vi "Dialog_Confirm Tling Parameters.vi"(0 "x FOV":dbl format="%#_3p", 5 "y FOV":dbl format="%#_3p", 9 "actual \noverlap\npercentage":dbl format="%#_3g", 11 "Error In":errorcluster, 12 "Tiling Rows":dbl, 13 "Tiling Columns":dbl) -> (6 "Cancelled?":bool, 15 "Error Out":errorcluster)   [LabVIEW 2012]
doc: "SciScan 1.2 160622\nThis VI has no controls.\nThis is a dummy whihc runs when user selects a macro command which does not require any arguments"
panel:
  in  "Cancel Button":bool
  in  "OK Button":bool
  # "Please confirm total FOV and number of rows & columns. \nActual overlap percentage is calculated based on the FOV \nsize of each individual tile (as configured in the main GUI)"
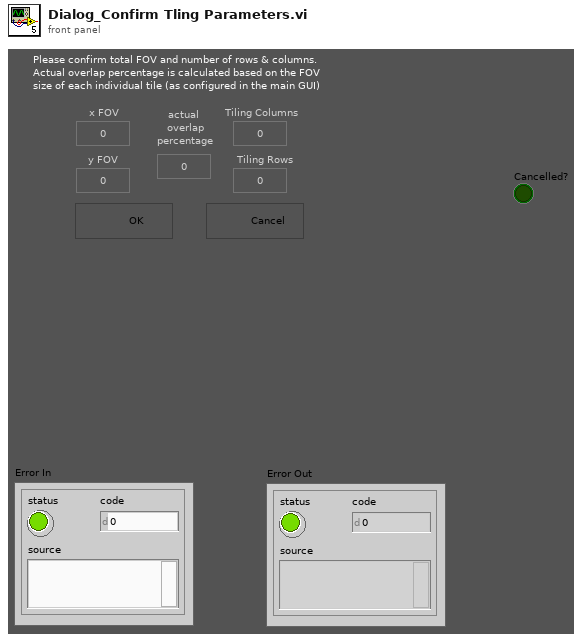
[diagram p1: front panel]
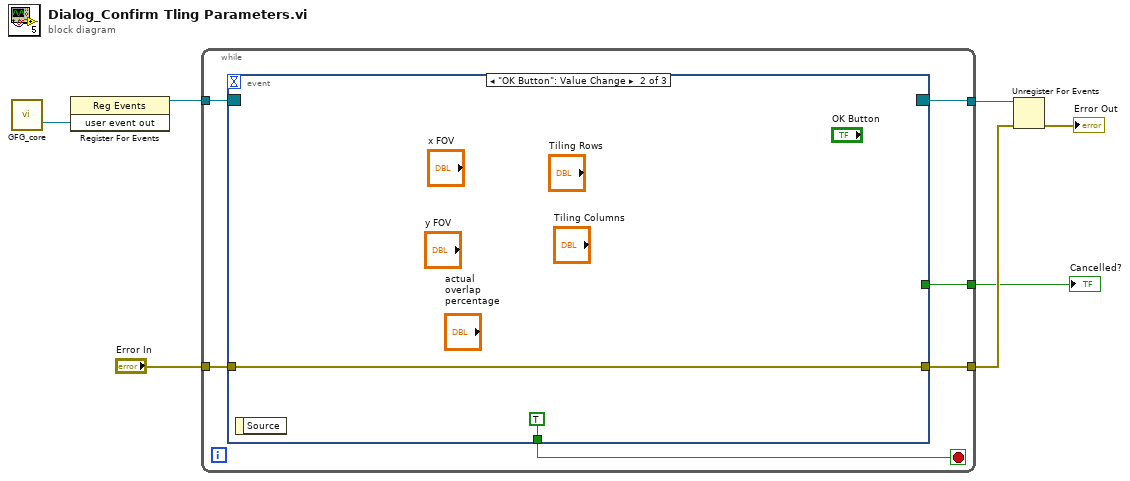
[diagram p0: block diagram]
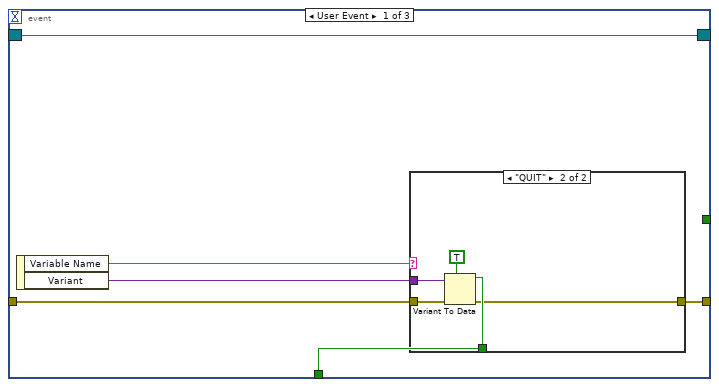
[diagram p2: hidden frame]
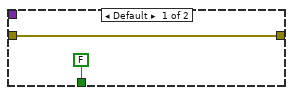
[diagram p3: hidden frame]
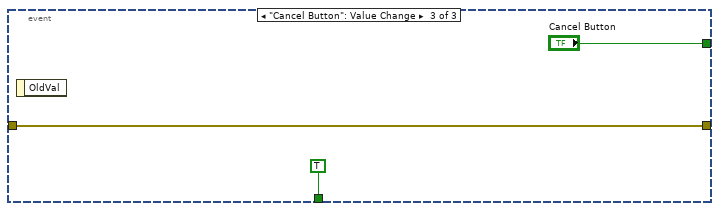
[diagram p4: hidden frame]
diagram:
  n1 = call "GFG_core.vi"() -> ("user event out"=w7:refnum<user-event>)  [unwired: 13 in, 6 out]
  n2 = register-events(w7) -> (reference out=w6:refnum<event-registration>)  [unwired: 2 in, 1 out]
  n3 = while {
    tunnel: w6 -> [w13]
    tunnel: [w12] -> w5
    tunnel: "Error In" -> [w10]
    tunnel: [w9] -> w3
    tunnel: [w8] -> w1
    stop <- w11 stop-if-true
    n4 = event shown="[1] \"OK Button\": Value Change" {
      selector: w13 -> [w19 _ _]
      dyn-events: [w19 _ _] -> w12
      timeout: _ -> [_ _ _]
      tunnel: [w16 TRUE TRUE] -> w11
      tunnel: w10 -> [w15 w27 w30]
      tunnel: [w14 w27 w30] -> w9
      tunnel: [_ _ "Cancel Button"] -> w8
      event User Event {
        n5 = event-data() -> ("Variable Name"=w18:string, "Variant"=w17:variant)  [unwired: 1 in]
        n6 = case shown="\"QUIT\"" w18 {
          tunnel: w17 -> [_ w25]
          tunnel: [FALSE w24] -> w16
          tunnel: w15 -> [w20 w23]
          tunnel: [w20 w22] -> w14
          frame Default {
          }
          frame "QUIT" {
            n7 = Variant To Data(error in=w23, type=TRUE, Variant=w25) -> (data=w24:bool, error out=w22:errorcluster)
          }
        }
      }
      event "OK Button": Value Change {
        n8 = event-data() -> ()  [unwired: 1 in, 1 out]
      }
      event "Cancel Button": Value Change {
        n9 = event-data() -> ()  [unwired: 1 in, 1 out]
      }
    }
  }
  "Cancelled?" <- w1
  n10 = Unregister For Events(event registration refnum=w5, error in=w3) -> (error out=→"Error Out":errorcluster)
